vi "MW_Display_Py_Open.vi"(0 "Env path":path=path "D:/dev/Guy_Storage/.venv", 5 "Python version":string="3.12", 11 "error in":errorcluster) -> (4 "session out":refnum<k35>, 15 "error out":errorcluster)   [LabVIEW 2023]
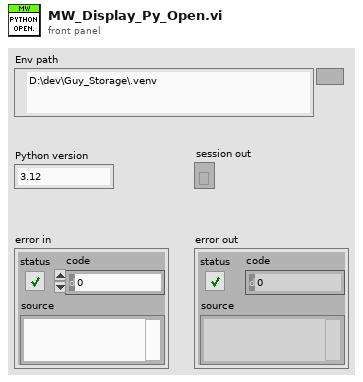
[diagram p1: front panel]
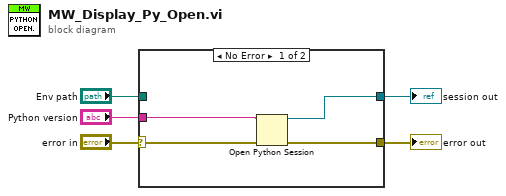
[diagram p0: block diagram]
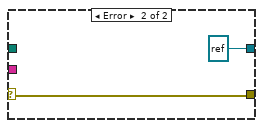
[diagram p2: hidden frame]
diagram:
  n1 = case shown="No Error" "error in" {
    selector: "error in" -> [w7 w11]
    tunnel: "Env path" -> [_ _]
    tunnel: "Python version" -> [w6 _]
    tunnel: [w9 refnum<k35> refnum ("session out")] -> w3
    tunnel: [w8 w11] -> w2
    frame No Error {
      n2 = Open Python Session(python version=w6, 3:w7) -> (session out=w9:refnum<k35>, error out=w8:errorcluster)  [unwired: 1 in]
    }
    frame Error {
    }
  }
  "session out" <- w3
  "error out" <- w2
